vi "KundtsTube.vi"() -> ()   [LabVIEW 2015]
uses:
  <vilib>/Utility/file.llb/Write Delimited Spreadsheet (DBL).vi
panel:
  out "Numeric":i32=49
  out "XY Graph":cluster{dbl[], dbl[]}(graph)={[10.0, 213.87755102040816, 417.7551020408163, 621.6326530612245, 825.5102040816327, 1029.3877551020407, 1233.265306122449, 1437.142857142857, 1641.0204081632653, 1844.8979591836735, 2048.7755102040815, 2252.6530612244896, 2456.530612244898, 2660.408163265306, 2864.285714285714, 3068.1632653061224, 3272.0408163265306, 3475.918367346939, 3679.795918367347, 3883.673469387755, 4087.5510204081634, 4291.428571428572, 4495.306122448979, 4699.183673469388, 4903.061224489796, 5106.938775510204, 5310.816326530612, 5514.693877551021, 5718.571428571428, 5922.448979591837, 6126.326530612245, 6330.2040816326535, 6534.081632653061, 6737.959183673469, 6941.836734693878, 7145.714285714285, 7349.591836734694, 7553.469387755102, 7757.34693877551, 7961.224489795918, 8165.102040816327, 8368.979591836734, 8572.857142857143, 8776.734693877552, 8980.612244897959, 9184.489795918367, 9388.367346938776, 9592.244897959185, 9796.122448979591, 10000.0], [-62.17108978559706, -62.75643978628702, -49.71123215814656, -54.102229934820436, -51.90116598952198, -32.65447945298821, -48.44071170937476, -53.137602710342705, -53.71790847670653, -47.290485636626656, -51.924532901046945, -53.49825960589101, -56.88625217792912, -56.704070948274186, -47.98443778155446, -56.36619454372756, -54.19840769213892, -54.75742286088354, -49.94362232194902, -60.61537255882891, -54.68990813232507, -54.05035376431054, -53.79764313946282, -60.887227612392024, -56.31601078540464, -54.82196752673549, -55.07890515301149, -60.750155650110884, -55.39826776230575, -54.733180663970096, -55.33153668765878, -61.71656847796, -54.916327419386434, -54.55591740334768, -54.29842469099228, -59.540141407331646, -55.15494653431068, -57.09058373191396, -56.18094354611056, -54.9618424959796, -58.60910088294797, -62.39906847679774, -62.70970190950723, -56.067154915224904, -59.63683798264646, -53.14947666041266, -54.368487349225745, -60.899121025521595, -54.96911583374481, -58.12613638010881]}
  out "Frequency":dbl=10000.0
  out "Waveform Graph":dynamicdata(graph)=[{"t0"=timestamp(3530054183.45926 s since 1904-01-01), "dt"=9.999999999999972e-06, "Y"=array[100000 elements], "attributes"=variant("NI_ChannelName"=variant(string "Voltage"), "NI_UnitDescription"=variant(string "Volts"))}]
  out "RMS":dbl=0.0043868035626247115
  in  "Sample Rate (hz)":dbl=100000.0
  in  "Sample number":i32=100000
  in  "Amplitude":dbl=5.0
  in  "Minimum":i32=10
  in  "# of points":dbl=50.0
  in  "Maximum":dbl=10000.0
  in  "Spacing":enum16{"Linear", "Logarithmic", ""}(ring)
  in  "Tab Control":enum32{"Sweep", "Single"}(tab)
  in  "Dwell Time (ms)":u32=1000
  in  "Single Freq":dbl
  # "Begining and End frequencies had fair bit of noise, but rest of values were clear. Run function to confrim!"
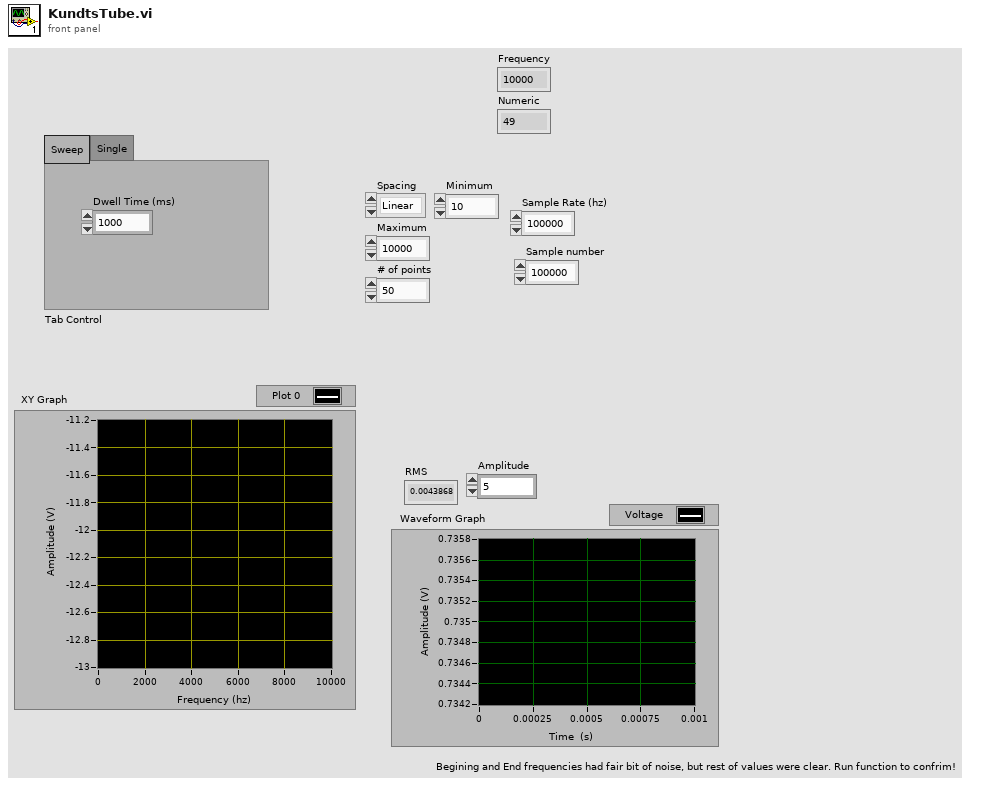
[diagram p1: front panel]
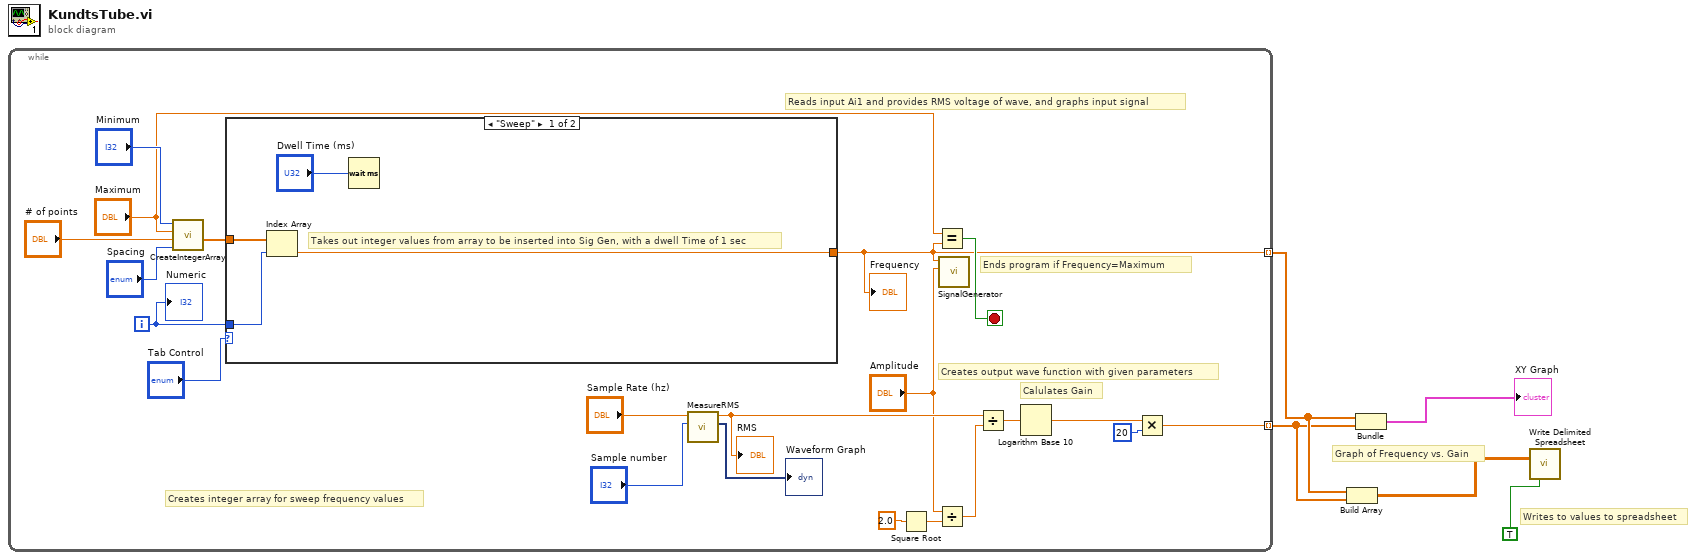
[diagram p0: block diagram]
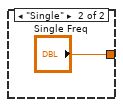
[diagram p2: hidden frame]
diagram:
  # "Writes to values to spreadsheet"
  # "Graph of Frequency vs. Gain"
  n1 = while {
    tunnel: [w18] -> w2 mode=indexing
    tunnel: [w6] -> w3 mode=indexing
    i -> [w10]
    stop <- w9 stop-if-true
    # "Calulates Gain"
    # "Creates integer array for sweep frequency values"
    # "Creates output wave function with given parameters"
    # "Ends program if Frequency=Maximum"
    # "Reads input Ai1 and provides RMS voltage of wave, and graphs input signal"
    n2 = call "CreateIntegerArray.vi"("Spacing"="Spacing", "# of points"="# of points", "Maximum"="Maximum", "Minimum"="Minimum") -> ("Frequency"=w11:dbl[])  [unwired: 7 in]
    n3 = case shown="\"Sweep\"" "Tab Control" {
      tunnel: [w29 "Single Freq"] -> w6
      tunnel: w10 -> [w30 _]
      tunnel: w11 -> [w28 _]
      frame "Sweep" {
        # "Takes out integer values from array to be inserted into Sig Gen, with a dwell Time of 1 sec"
        n4 = Index Array(array=w28, index=w30) -> (element=w29:dbl)
        n5 = Wait (ms)(milliseconds to wait="Dwell Time (ms)") -> ()  [unwired: 1 out]
      }
      frame "Single" {
      }
    }
    "Frequency" <- w6
    n6 = call "MeasureRMS.vi"("Sample number"="Sample number", "Sample Rate (hz)"="Sample Rate (hz)") -> ("Waveform Graph"=→"Waveform Graph":dynamicdata, "RMS"=w19:dbl)  [unwired: 8 in]
    "RMS" <- w19
    n7 = Square Root(x=2.0) -> (sqrt(x)=w17:dbl)
    n8 = Equal?(x="Maximum", y=w6) -> (x = y?=w9:bool)
    n9 = Divide(x="Amplitude", y=w17) -> (x/y=w15:dbl)
    n10 = call "SignalGenerator.vi"("Amplitude"="Amplitude", "Frequency"=w6) -> ()  [unwired: 9 in, 1 out]
    n11 = Divide(x=w19, y=w15) -> (x/y=w21:dbl)
    n12 = Logarithm Base 10(1:w21) -> (0:w20:dbl)
    n13 = Multiply(x=w20, y=20) -> (x*y=w18:dbl)
    "Numeric" <- w10
  }
  n14 = Build Array(w3, w2) -> (w4:dbl[][])
  n15 = Bundle(w3, w2) -> (→"XY Graph":cluster{dbl[], dbl[]})  [unwired: 1 in]
  n16 = call-poly <vilib>:"Write Delimited Spreadsheet.vi"("2D data"=w4, "transpose? (F)"=TRUE) -> ()  [unwired: 12 in, 2 out]
